vi "Compress.vi"(11 "Trace Items In":cluster{string, bool}[](array[cluster])) -> (1 "Active Compressed Out":string[](array[string]))   [LabVIEW 2018, in "TracerLibrary.lvlib" / "Tracer.lvclass"]
uses:
  Tracer.lvclass
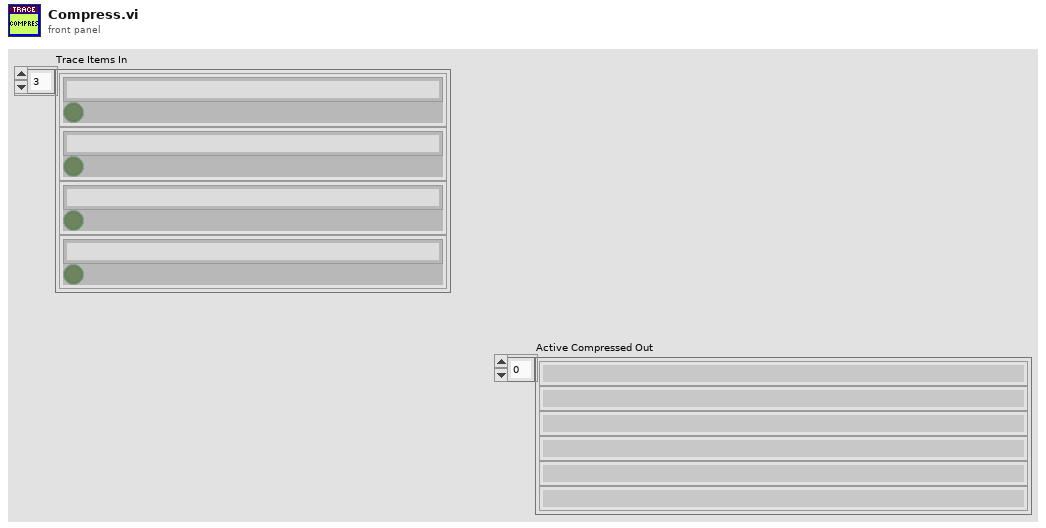
[diagram p1: front panel]
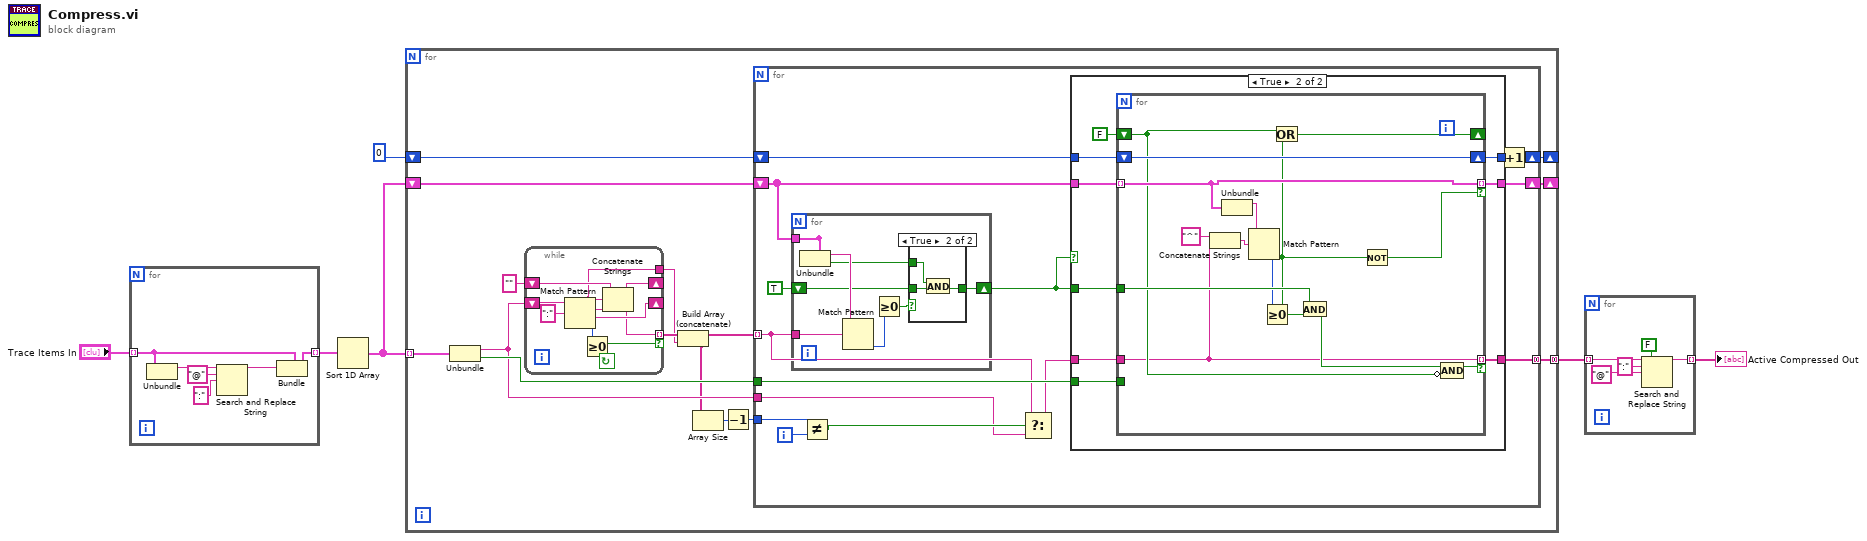
[diagram p0: block diagram]
diagram:
  n1 = for {
    tunnel: [w8] -> w4 mode=indexing
    tunnel: "Trace Items In" -> [w9] mode=indexing
    n2 = Unbundle(w9) -> (w10:string)  [unwired: 1 out]
    n3 = Search and Replace String(input string=w10, search string="@", replace string=":" ("search string")) -> (result string=w7:string)  [unwired: 5 in, 3 out]
    n4 = Bundle(cluster=w9, w7) -> (w8:cluster{string, bool})  [unwired: 1 in]
  }
  n5 = Sort 1D Array(array=w4) -> (sorted array=w6:cluster{string, bool}[])
  n6 = for {
    tunnel: w6 -> [w26] mode=indexing
    tunnel: [w22] -> w2 mode=concatenating
    shift-right: [w19] -> _
    shift-left: 0 -> [w20]
    shift-right: [w23] -> _
    shift-left: w6 -> [w18]
    n7 = Unbundle(w26) -> (w16:string, w24:bool)
    n8 = while {
      shift-right: [w83] -> _
      shift-left: w16 -> [w87]
      shift-right: [w82] -> _
      shift-left: "" -> [w84]
      tunnel: [w82] -> w21 mode=indexing if=w80
      tunnel: [w79] -> w17
      stop <- w80 continue-if-true
      n9 = Match Pattern(string=w87, regular expression=":") -> (before substring=w79:string, match substring=w85:string, after substring=w83:string, offset past match=w81:i32)  [unwired: 1 in]
      n10 = Greater Or Equal To 0?(x=w81) -> (x >= 0?=w80:bool)
      n11 = Concatenate Strings(w84, w79, w85) -> (w82:string)
    }
    n12 = Build Array (concatenate)(w21, w17) -> (w15:string[])
    n13 = Array Size(array=w15) -> (size(s)=w14:i32)
    n14 = Decrement(x=w14) -> (x-1=w13:i32)
    n15 = for {
      tunnel: w15 -> [w27] mode=indexing
      tunnel: w24 -> [w40]
      tunnel: [w38] -> w22 mode=concatenating
      shift-right: [w34] -> w19
      shift-left: w20 -> [w37]
      shift-right: [w39] -> w23
      shift-left: w18 -> [w33]
      tunnel: w16 -> [w29]
      tunnel: w13 -> [w31]
      i -> [w32]
      n16 = for {
        tunnel: w33 -> [w67] mode=indexing
        tunnel: w27 -> [w73]
        shift-right: [w70] -> w35
        shift-left: TRUE -> [w71]
        tunnel: [w67] -> _
        n17 = Unbundle(w67) -> (w74:string, w68:bool)
        n18 = Match Pattern(string=w74, regular expression=w73) -> (offset past match=w72:i32)  [unwired: 1 in, 3 out]
        n19 = Greater Or Equal To 0?(x=w72) -> (x >= 0?=w69:bool)
        n20 = case shown="True" w69 {
          tunnel: w71 -> [w75 w78]
          tunnel: [w75 w77] -> w70
          tunnel: w68 -> [_ w76]
          frame False {
          }
          frame True {
            n21 = And(x=w76, y=w78) -> (x .and. y?=w77:bool)
          }
        }
      }
      n22 = Not Equal?(x=w31, y=w32) -> (x != y?=w30:bool)
      n23 = Select(t=w27, s=w30, f=w29) -> (s? t:f=w28:string)
      n24 = case shown="True" w35 {
        tunnel: w40 -> [_ w52]
        tunnel: w35 -> [_ w51]
        tunnel: w28 -> [_ w50]
        tunnel: [w42 w49] -> w39
        tunnel: [_ w48] -> w38
        tunnel: w33 -> [w42 w46]
        tunnel: w37 -> [w43 w45]
        tunnel: [w43 w44] -> w36
        frame False {
        }
        frame True {
          n25 = for {
            tunnel: w52 -> [_]
            tunnel: w51 -> [w65]
            tunnel: w50 -> [w55]
            tunnel: [w55] -> w48 mode=indexing if=w62
            shift-right: [w56] -> _
            shift-left: FALSE -> [w58]
            shift-right: [w61] -> w44
            shift-left: w45 -> [w61]
            tunnel: w46 -> [w59] mode=indexing
            tunnel: [w59] -> w49 mode=indexing if=w60
            n26 = Concatenate Strings("^" ("string"), w55) -> (w54:string)
            n27 = Unbundle(w59) -> (w66:string)  [unwired: 1 out]
            n28 = Match Pattern(string=w66, regular expression=w54) -> (offset past match=w64:i32)  [unwired: 1 in, 3 out]
            n29 = Greater Or Equal To 0?(x=w64) -> (x >= 0?=w57:bool)
            n30 = Or(x=w58, y=w57) -> (x .or. y?=w56:bool)
            n31 = And(x=w65, y=w57) -> (x .and. y?=w63:bool)
            n32 = Not(x=w57) -> (.not. x?=w60:bool)
            n33 = Compound Arithmetic op=AND(w63, invert w58) -> (w62:bool)
          }
        }
      }
      n34 = Increment(x=w36) -> (x+1=w34:i32)
    }
  }
  n35 = for {
    tunnel: w2 -> [w92] mode=indexing
    tunnel: [w88] -> w1 mode=indexing
    n36 = Search and Replace String(replace all?=FALSE ("replace all? (F)"), input string=w92, search string=":", replace string="@" ("search string")) -> (result string=w88:string)  [unwired: 4 in, 3 out]
  }
  "Active Compressed Out" <- w1
